vi "Untitled 1.vi"() -> ()   [LabVIEW 2025]
panel:
  out "x-y":u32
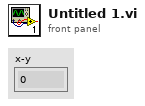
[diagram p1: front panel]
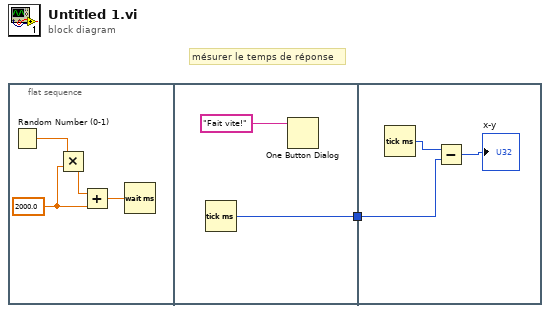
[diagram p0: block diagram]
diagram:
  # "mésurer le temps de réponse"
  n1 = flat-sequence {
    tunnel: [w6] -> w1
    tunnel: w1 -> [w8]
    frame #0 {
      w2 = 2000.0 ("y")
      n2 = Random Number (0-1)() -> (number: 0 to 1=w5:dbl)
      n3 = Multiply(x=w5, y=w2) -> (x*y=w3:dbl)
      n4 = Add(x=w3, y=w2) -> (x+y=w4:dbl)
      n5 = Wait (ms)(milliseconds to wait=w4) -> ()  [unwired: 1 out]
    }
    frame #1 {
      n6 = Tick Count (ms)() -> (millisecond timer value=w6:u32)
      n7 = One Button Dialog(message="Fait vite!") -> ()  [unwired: 1 in, 1 out]
    }
    frame #2 {
      n8 = Tick Count (ms)() -> (millisecond timer value=w9:u32)
      n9 = Subtract(x=w9, y=w8) -> (x-y=→"x-y":u32)
    }
  }
